vi "readAutonCSV.vi"(2 "AutonFile":string) -> (6 "AutonArray":dbl[][](array[numeric]))   [LabVIEW 2011]
doc: "Use this VI to read comma delimited text files for input of autonomous data. Data should be in rows, in the following order: 1) Primitive ID number, 2) Heading (deg), 3) time(s)/Dist(in), 4) Power."
uses:
  <vilib>/Utility/file.llb/Read From Spreadsheet File (DBL).vi
panel:
  out "Path and file":string
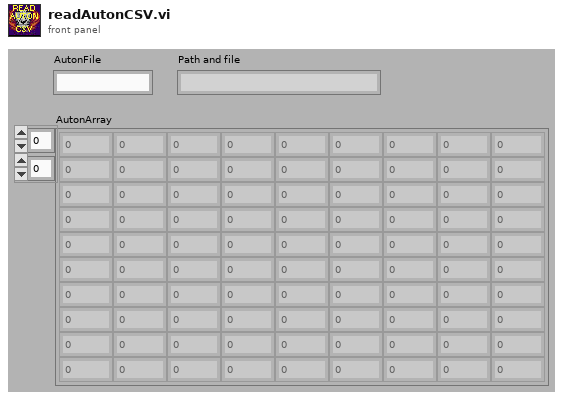
[diagram p1: front panel]
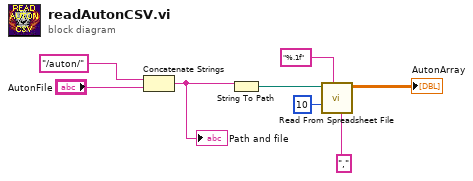
[diagram p0: block diagram]
diagram:
  n1 = Concatenate Strings("/auton/" ("string"), "AutonFile") -> (w3:string)
  "Path and file" <- w3
  n2 = String To Path(string=w3) -> (path=w2:path)
  n3 = call-poly <vilib>:"Read From Spreadsheet File.vi"("delimiter (\\t)"="," ("delimiter (\\t)"), "format (%.3f)"="%.1f", "number of rows (all:-1)"=10, "file path (dialog if empty)"=w2) -> ("all rows"=→"AutonArray":dbl[][])  [unwired: 1 in, 6 out]
